vi "ABOUT SCREEN ADV NEW.vi"(8 "error in (no error)":errorcluster, 11 "Array":string[](array[string])) -> (0 "error out":errorcluster)   [LabVIEW 2025]
uses:
  <vilib>/Utility/traverseref.llb/TRef TravTarget.ctl
  <vilib>/Utility/traverseref.llb/VI Scripting - Traverse.lvlib
panel:
  out "version":string="v1.AU.26"
  out "reference out":refnum<vi>
  in  "close":bool
  in  "Tab Selection":enum32{"About", "License", "Company"}(radio) caption="Radio Buttons - Customizable"
  out "Tab Control":T1(tab)
  out "Operating System":string="Windows 11 Pro"
  out "Version":string="1.AU.26"
  out "Workorder":string="2479"
  out "Runtime":string="LabVIEW 2025 (64-bit)"
  out "Instrument Serial":string="770073"
  out "Firmware Version":string="BCLV 3.6"
  # "v"
  # "© Copyright 2023 | Paltro Inc."
  # "All rights reserved."
  # "Version"
  # "Workorder"
  # "Runtime"
  # "Copyright"
  # "© 2023"
  # "Firmware Version"
  # "Operating System"
  # "Instrument Serial"
  # "Status"
  # "."
  # "Active"
  # "Licence Type"
  # "Single-seat commercial"
  # "Seats"
  # "1 of 1 in use"
  # "Expires"
  # "Perpetual"
  # "URL"
  # "Company"
  # "hello@palto.com"
  # "Mail"
  # "https://www.paltro.com"
  # "Website"
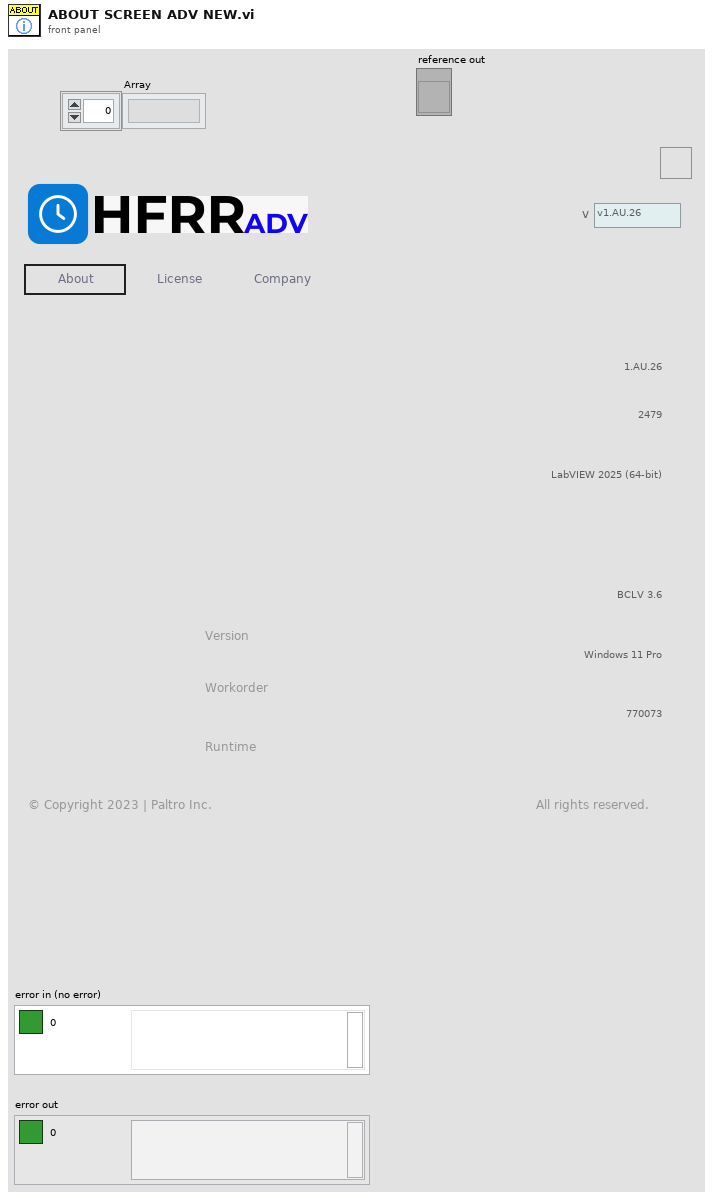
[diagram p1: front panel]
types:
  T1 = enum32{"About", "License", "Company", "System info"}
  T2 = typedef "TRef TravTarget.ctl" = enum16{"FP", "BD", "Other"}
  T3 = enum32{"Invalid", "Standard", "Closed", "Hidden", "Minimized", "Maximized"}
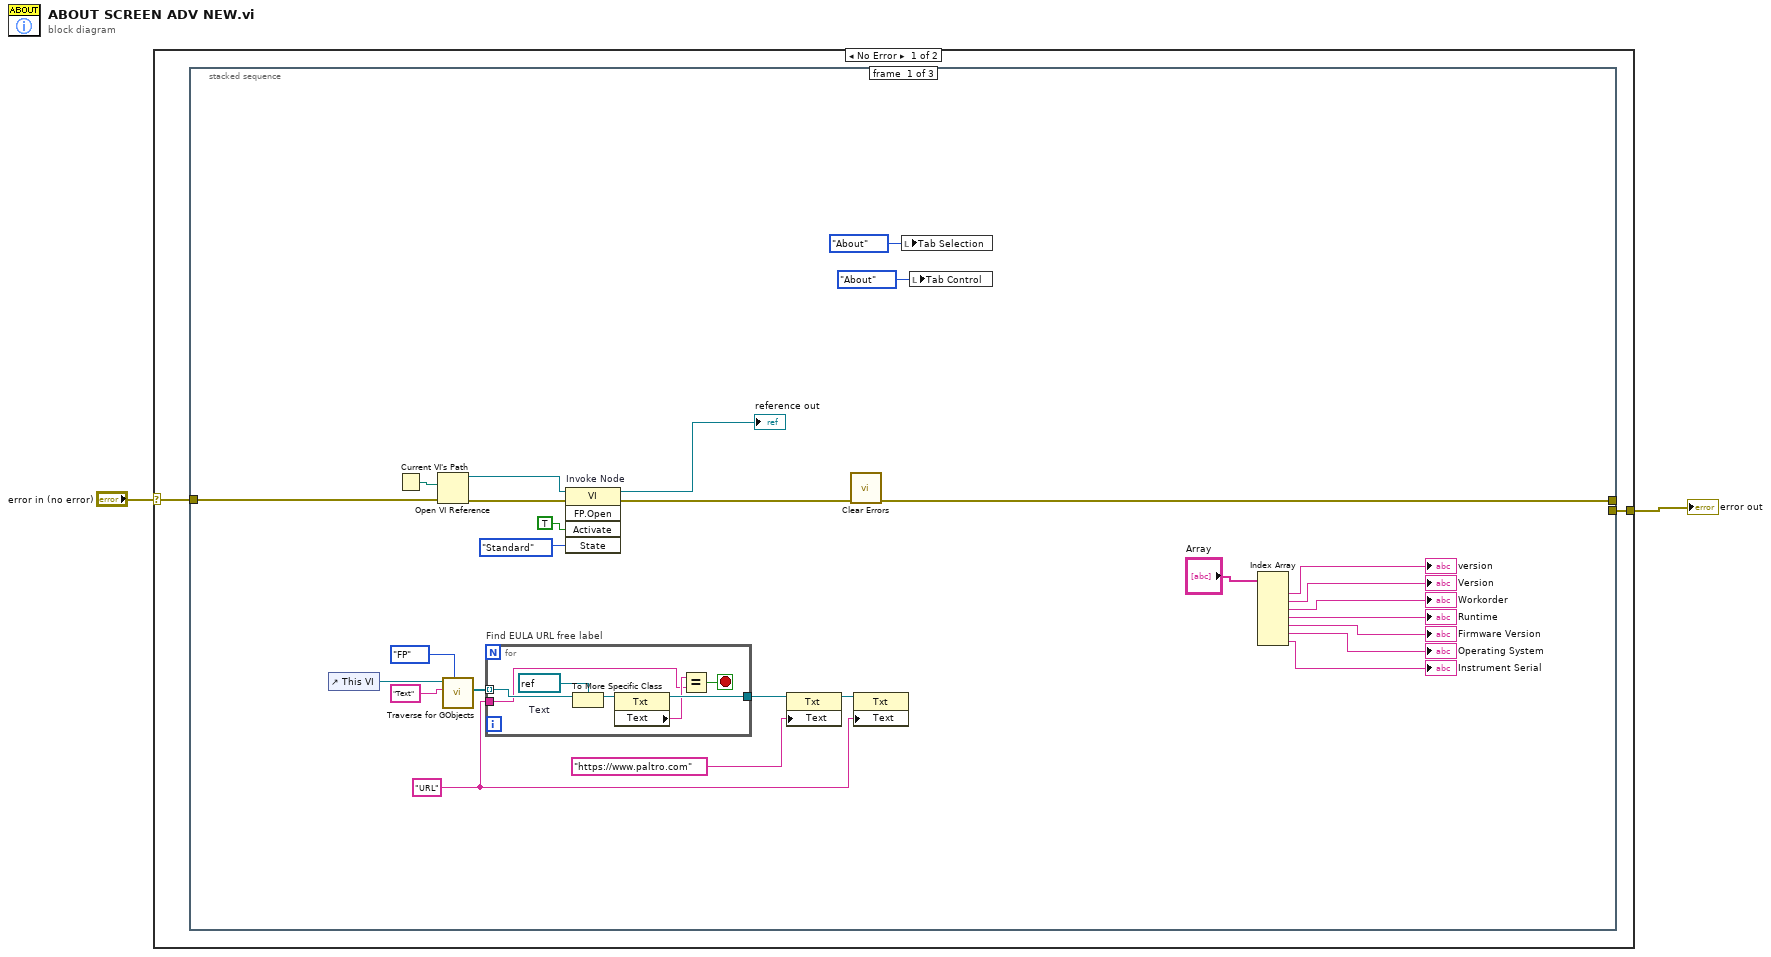
[diagram p0: block diagram]
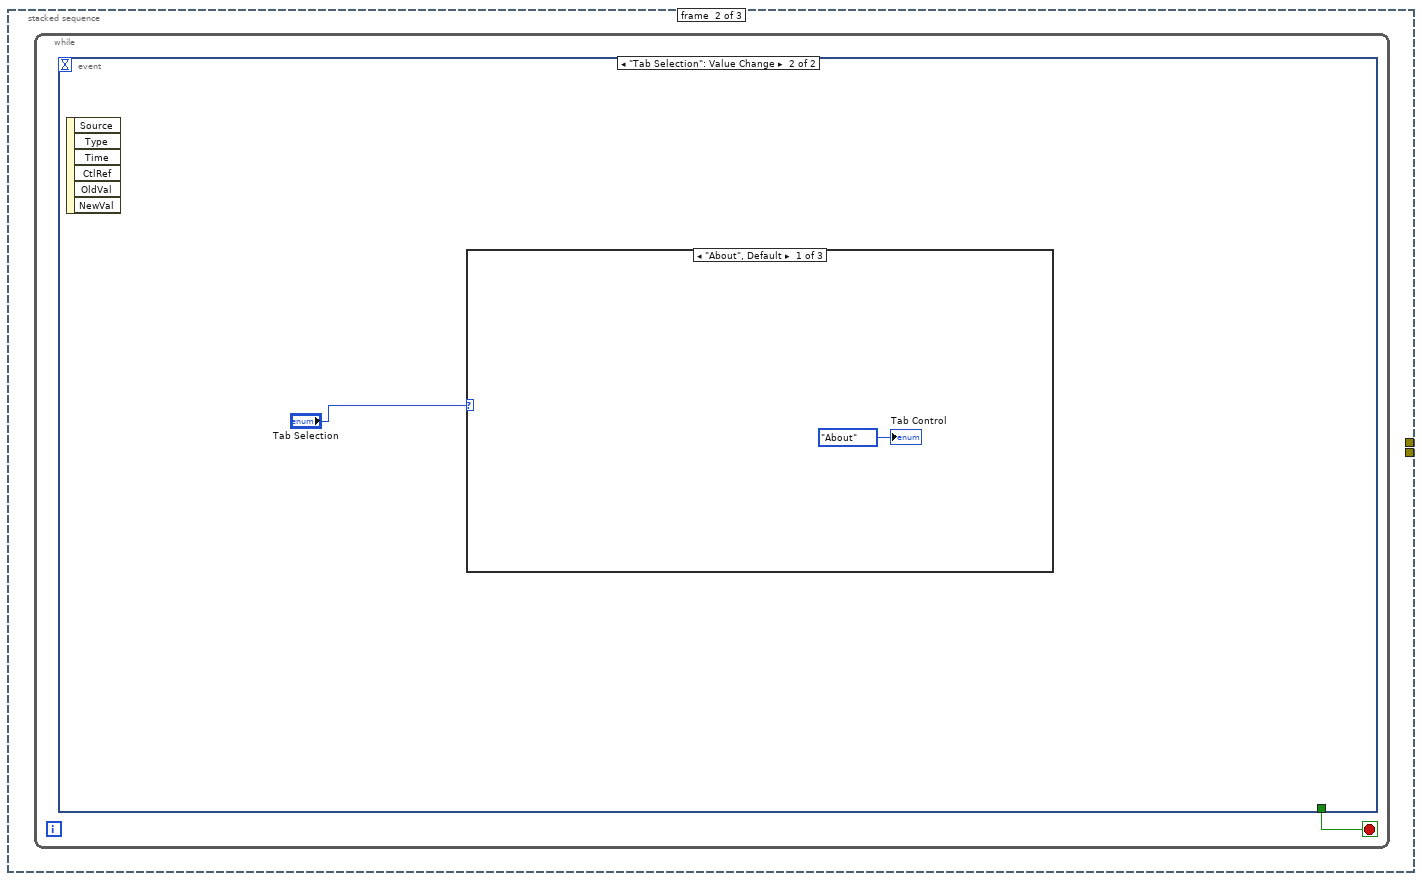
[diagram p2: hidden frame]
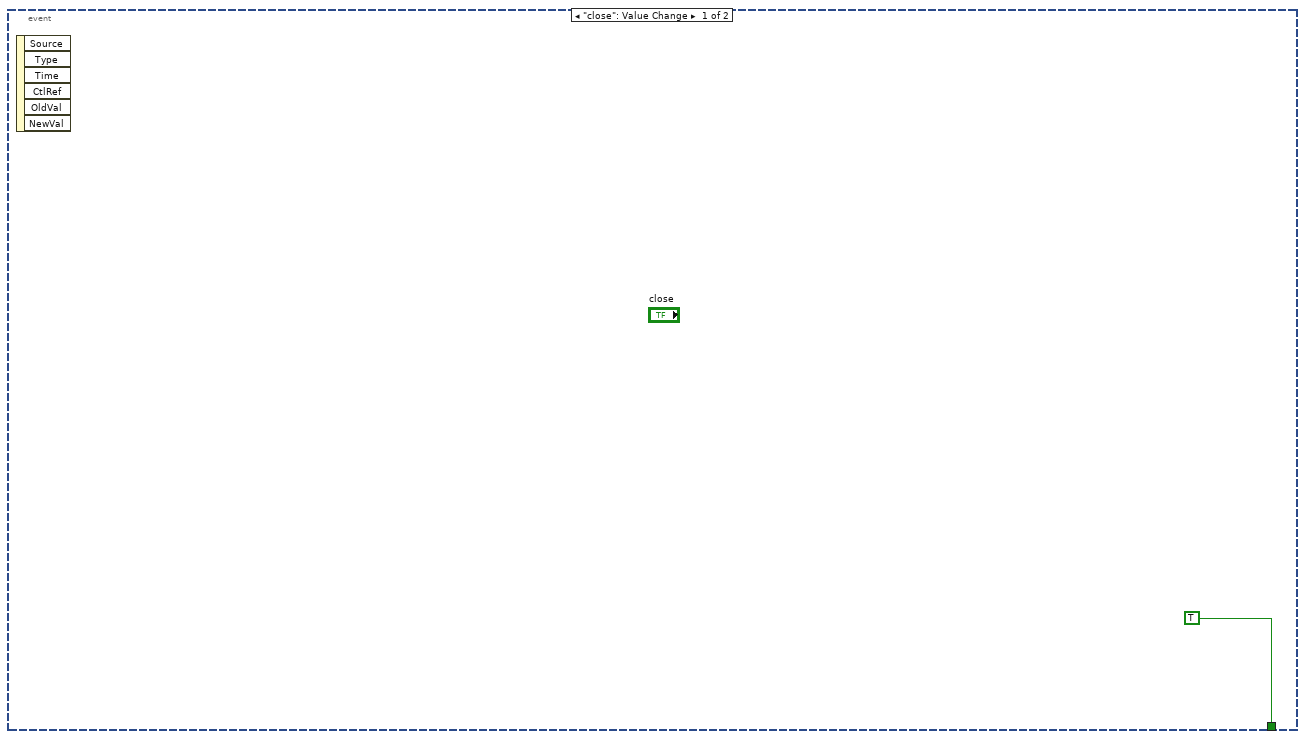
[diagram p3: hidden frame]
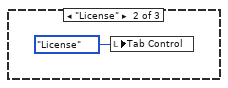
[diagram p4: hidden frame]
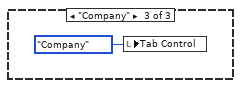
[diagram p5: hidden frame]
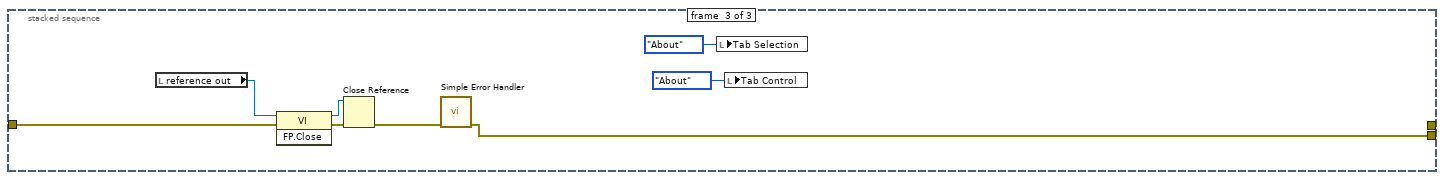
[diagram p6: hidden frame]
diagram:
  n1 = case shown="No Error" "error in (no error)" {
    selector: "error in (no error)" -> [w4 _]
    tunnel: [w3 _] -> w1
    frame No Error {
      n2 = stacked-sequence {
        tunnel: w4 -> [w26 _ w49]
        tunnel: [w21 _ _] -> _
        tunnel: [_ _ w47] -> w3
        frame #0 {
          w17 = "URL"
          n3 = control-ref of="This VI"() -> (w14:refnum<vi>)
          n4 = Current VI's Path() -> (path=w31:path)
          n5 = Open VI Reference(vi path=w31, error in (no error)=w26) -> (vi reference=w27:refnum<vi>, error out=w28:errorcluster)  [unwired: 4 out]
          n6 = call <vilib>:"Traverse for GObjects.vi"("Traverse Target"=TRef_TravTarget."FP", "Class Name"="Text", "VI Refnum"=w14) -> ("References"=w12:refnum<vi>[])  [unwired: 5 in, 3 out]
          n7 = for "Find EULA URL free label" {
            tunnel: w12 -> [w38] mode=indexing
            tunnel: [w35] -> w11
            tunnel: w17 -> [w33]
            stop <- w32 stop-if-true
            w37 = refnum<vi> refnum  # Text
            n8 = To More Specific Class(target class=w37, reference=w38) -> (specific class reference=w36:refnum<vi>)  [unwired: 1 in, 1 out]
            n9 = property class="Txt"(reference=w36) -> (reference out=w35:refnum<vi>, "Text"=w34:string)  [unwired: 1 in, 1 out]
            n10 = Equal?(x=w34, y=w33) -> (x = y?=w32:bool)
          }
          n11 = invoke on="Invoke Node" class="VI" method="FP.Open"(reference=w27, error in=w28, "Activate"=TRUE ("Activate?"), "State"=T3."Standard") -> (reference out=→"reference out":refnum<vi>, error out=w25:errorcluster)  [unwired: 1 in, 3 out]
          n12 = property class="Txt"(reference=w11, "Text"="https://www.paltro.com") -> (reference out=w16:refnum<vi>)  [unwired: 1 in, 1 out]
          n13 = call <vilib>:"Clear Errors.vi"("error in (no error)"=w25) -> ("error out"=w21:errorcluster)  [unwired: 5 in, 1 out]
          n14 = property class="Txt"(reference=w16, "Text"=w17) -> ()  [unwired: 1 in, 2 out]
          n15 = local write "Tab Selection"(enum32{"About", "License", "Company"}."About" ("Tab Selection")) -> ()
          n16 = local write "Tab Control"(T1."About" ("Tab Control")) -> ()
          n17 = Index Array(array="Array") -> (element #1=→"version":string, element #2=→"Version":string, element #3=→"Workorder":string, element #4=→"Runtime":string, element #5=→"Firmware Version":string, element #6=→"Operating System":string, element #7=→"Instrument Serial":string)  [unwired: 7 in]
        }
        frame #1 {
          n18 = while {
            stop <- w39 stop-if-true
            n19 = event shown="[1] \"Tab Selection\": Value Change" {
              selector: _ -> [_ _]
              dyn-events: _ -> [_ _]
              timeout: _ -> [_ _]
              tunnel: [TRUE _] -> w39
              event "close": Value Change {
                n20 = event-data() -> ()  [unwired: 1 in, 6 out]
              }
              event "Tab Selection": Value Change {
                n21 = event-data() -> ()  [unwired: 1 in, 6 out]
                n22 = case shown="\"About\", Default" "Tab Selection" {
                  frame "About", Default {
                    "Tab Control" <- T1."About" ("Tab Control")
                  }
                  frame "License" {
                    n23 = local write "Tab Control"(T1."License" ("Tab Control")) -> ()
                  }
                  frame "Company" {
                    n24 = local write "Tab Control"(T1."Company" ("Tab Control")) -> ()
                  }
                }
              }
            }
          }
        }
        frame #2 {
          n25 = local read "reference out"() -> (w48:refnum<vi>)
          n26 = invoke class="VI" method="FP.Close"(reference=w48, error in=w49) -> (reference out=w51:refnum<vi>, error out=w52:errorcluster)  [unwired: 1 in, 1 out]
          n27 = Close Reference(reference=w51, error in (no error)=w52) -> (error out=w50:errorcluster)
          n28 = call <vilib>:"Simple Error Handler.vi"("error in (no error)"=w50) -> ("error out"=w47:errorcluster)  [unwired: 1 in, 7 out]
          n29 = local write "Tab Selection"(enum32{"About", "License", "Company"}."About" ("Tab Selection")) -> ()
          n30 = local write "Tab Control"(T1."About" ("Tab Control")) -> ()
        }
      }
    }
    frame Error {
    }
  }
  "error out" <- w1
